vi "1337.vi"() -> ()   [LabVIEW 2010]
panel:
  out "x+y":i32
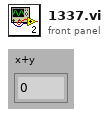
[diagram p1: front panel]
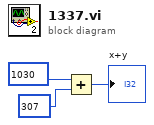
[diagram p0: block diagram]
diagram:
  n1 = Add(x=1030, y=307) -> (x+y=→"x+y":i32)
